vi "Tree.vi"() -> ()   [LabVIEW 2016, in "DAQ.lvclass"]
uses:
  SMOs/DAQ/DAQ.lvclass
  SMOs/DAQ/Typedefs/PublicEvents--DAQ.Read.ctl
  SMOs/DAQ/Typedefs/DAQ_Config.ctl
  SMOs/DAQ/Typedefs/PrivateEvents--DAQ.AI.Channels.ctl
  SMOs/DAQ/Typedefs/DAQ_Type.ctl
  SMOs/DAQ/Typedefs/DAQ_SamplingInfo.ctl
  SMOs/DAQ/Typedefs/DAQ_SamplingMode.ctl
panel:
  in  "Read 2":T1
  out "Read":T1
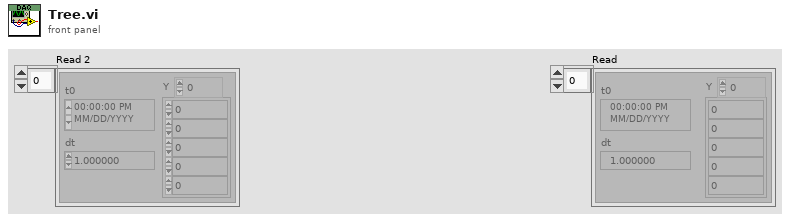
[diagram p1: front panel]
types:
  T1 = typedef "DAQ.lvclass/PublicEvents--DAQ.Read.ctl" = waveform(dbl)[]
  T2 = typedef "DAQ.lvclass/DAQ_Config.ctl" = cluster{"Channels":T3, "DAQ_Type":T4, "minimum value":dbl, "maximum value":dbl, "DAQ_SamplingInfo":T5, "DAQ_SamplingMode":T6}
  T3 = typedef "DAQ.lvclass/PrivateEvents--DAQ.AI.Channels.ctl" = string
  T4 = typedef "DAQ.lvclass/DAQ_Type.ctl" = enum16{"AI", "AO"}
  T5 = typedef "DAQ.lvclass/DAQ_SamplingInfo.ctl" = cluster{"Fs":dbl, "#s":i32}
  T6 = typedef "DAQ.lvclass/DAQ_SamplingMode.ctl" = enum16{"Continuous", "Finite"}
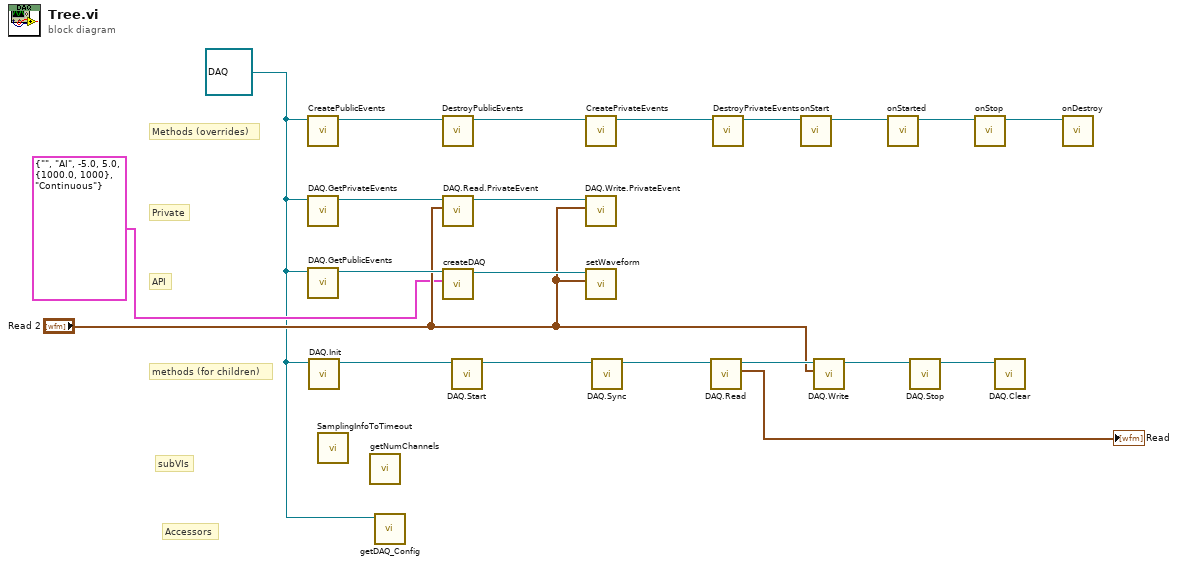
[diagram p0: block diagram]
diagram:
  w1 = refnum<class "DAQ.lvclass"> refnum ("DAQ.lvclass")
  # "Accessors"
  # "subVIs"
  # "methods (for children)"
  # "API"
  # "Private"
  # "Methods (overrides)"
  n1 = call-dynamic "CreatePublicEvents.vi"("DAQ"=w1) -> ("DAQ out"=w21:refnum<class "DAQ.lvclass">)  [unwired: 9 in, 1 out]
  n2 = call "DAQ.GetPrivateEvents.vi"("DAQ"=w1) -> ("DAQ out"=w14:refnum<class "DAQ.lvclass">)  [unwired: 8 in, 2 out]
  n3 = call "DAQ.GetPublicEvents.vi"("DAQ"=w1) -> ("DAQ out"=w12:refnum<class "DAQ.lvclass">)  [unwired: 8 in, 2 out]
  n4 = call-dynamic "DAQ.Init.vi"("DAQ in"=w1) -> ("DAQ out"=w10:refnum<class "DAQ.lvclass">)  [unwired: 9 in, 1 out]
  n5 = call "SamplingInfoToTimeout.vi"() -> ()  [unwired: 9 in, 2 out]
  n6 = call "getNumChannels.vi"() -> ()  [unwired: 9 in, 3 out]
  n7 = call "getDAQ_Config.vi"("DAQ in"=w1) -> ()  [unwired: 8 in, 3 out]
  n8 = call-dynamic "DestroyPublicEvents.vi"("DAQ"=w21) -> ("DAQ out"=w20:refnum<class "DAQ.lvclass">)  [unwired: 9 in, 1 out]
  n9 = call "DAQ.Read.PrivateEvent.vi"("DAQ.Read"="Read 2", "DAQ"=w14) -> ("DAQ out"=w13:refnum<class "DAQ.lvclass">)  [unwired: 8 in, 1 out]
  n10 = call "createDAQ.vi"("DAQ.Config"=T2 {"Channels"="", "DAQ_Type"=enum."AI", "minimum value"=-5.0, "maximum value"=5.0, "DAQ_SamplingInfo"={"Fs"=1000.0, "#s"=1000}, "DAQ_SamplingMode"=enum."Continuous"}, "DAQ in"=w12) -> ("DAQ out"=w11:refnum<class "DAQ.lvclass">)  [unwired: 8 in, 1 out]
  n11 = call-dynamic "DAQ.Start.vi"("DAQ in"=w10) -> ("DAQ out"=w9:refnum<class "DAQ.lvclass">)  [unwired: 9 in, 1 out]
  n12 = call-dynamic "CreatePrivateEvents.vi"("DAQ"=w20) -> ("DAQ out"=w19:refnum<class "DAQ.lvclass">)  [unwired: 9 in, 1 out]
  n13 = call "DAQ.Write.PrivateEvent.vi"("DAQ.Write"="Read 2", "DAQ"=w13) -> ()  [unwired: 8 in, 2 out]
  n14 = call "setWaveform.vi"("setWaveform"="Read 2", "DAQ"=w11) -> ()  [unwired: 8 in, 2 out]
  n15 = call-dynamic "DAQ.Sync.vi"("DAQ in"=w9) -> ("DAQ out"=w8:refnum<class "DAQ.lvclass">)  [unwired: 9 in, 1 out]
  n16 = call-dynamic "DAQ.Read.vi"("DAQ in"=w8) -> ("Read"=→"Read":waveform(dbl)[], "DAQ out"=w7:refnum<class "DAQ.lvclass">)  [unwired: 8 in, 1 out]
  n17 = call-dynamic "DestroyPrivateEvents.vi"("DAQ"=w19) -> ("DAQ out"=w18:refnum<class "DAQ.lvclass">)  [unwired: 9 in, 1 out]
  n18 = call-dynamic "onStart.vi"("DAQ"=w18) -> ("DAQ out"=w17:refnum<class "DAQ.lvclass">)  [unwired: 9 in, 1 out]
  n19 = call-dynamic "DAQ.Write.vi"("Write"="Read 2", "DAQ in"=w7) -> ("DAQ out"=w6:refnum<class "DAQ.lvclass">)  [unwired: 7 in, 2 out]
  n20 = call-dynamic "onStarted.vi"("SMO"=w17) -> ("SMO out"=w16:refnum<class "DAQ.lvclass">)  [unwired: 9 in, 1 out]
  n21 = call-dynamic "DAQ.Stop.vi"("DAQ in"=w6) -> ("DAQ out"=w5:refnum<class "DAQ.lvclass">)  [unwired: 9 in, 1 out]
  n22 = call-dynamic "onStop.vi"("DAQ"=w16) -> ("DAQ out"=w15:refnum<class "DAQ.lvclass">)  [unwired: 9 in, 1 out]
  n23 = call-dynamic "DAQ.Clear.vi"("DAQ in"=w5) -> ()  [unwired: 9 in, 2 out]
  n24 = call-dynamic "onDestroy.vi"("DAQ"=w15) -> ()  [unwired: 9 in, 2 out]
